vi "FGV_Counter.vi"(7 "Action (read)":T1=enum."Read", 8 "error in (no error)":errorcluster) -> (0 "error out":errorcluster, 3 "Counter":i32)   [LabVIEW 2020]
uses:
  #typedel_FGV_action.ctl
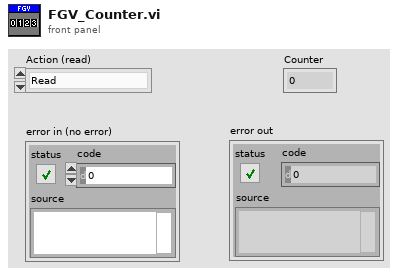
[diagram p1: front panel]
types:
  T1 = typedef "#typedel_FGV_action.ctl" = enum16{"Initialize", "Increment", "Decrement", "Read"}
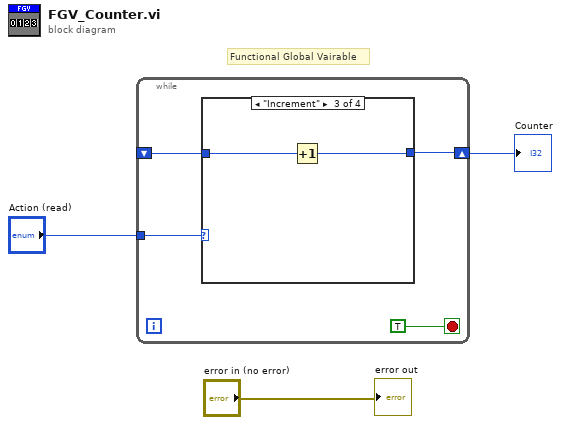
[diagram p0: block diagram]
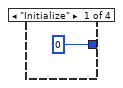
[diagram p2: hidden frame]
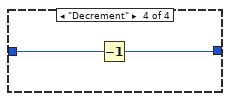
[diagram p4: hidden frame]
diagram:
  # "Functional Global Vairable"
  n1 = while {
    shift-right: [w5] -> w3
    shift-left: _ -> [w4]
    tunnel: "Action (read)" -> [w6]
    stop <- TRUE stop-if-true
    n2 = case shown="\"Increment\"" w6 {
      tunnel: [0 w9 w10 w12] -> w5
      tunnel: w4 -> [_ w9 w11 w13]
      frame "Initialize" {
      }
      frame "Read", Default {
      }
      frame "Increment" {
        n3 = Increment(x=w11) -> (x+1=w10:i32)
      }
      frame "Decrement" {
        n4 = Decrement(x=w13) -> (x-1=w12:i32)
      }
    }
  }
  "Counter" <- w3
  "error out" <- "error in (no error)"
